vi "Init TS User Events.vi"(8 "error in (no error)":errorcluster, 11 "Generic Test Stand in":refnum<class "Generic Test Stand.lvclass">) -> (0 "error out":errorcluster, 3 "Generic Test Stand out":refnum<class "Generic Test Stand.lvclass">)   [LabVIEW 2019, in "Generic Test Stand.lvclass"]
uses:
  Generic Test Stand.lvclass
  Generic Test Stand.lvclass/Generic Test Stand.ctl
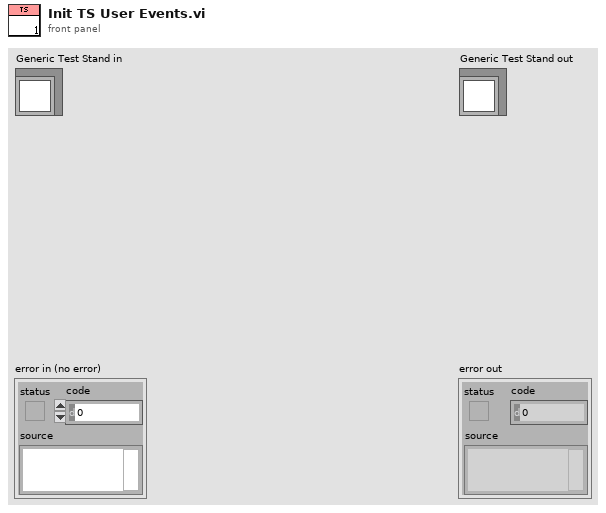
[diagram p1: front panel]
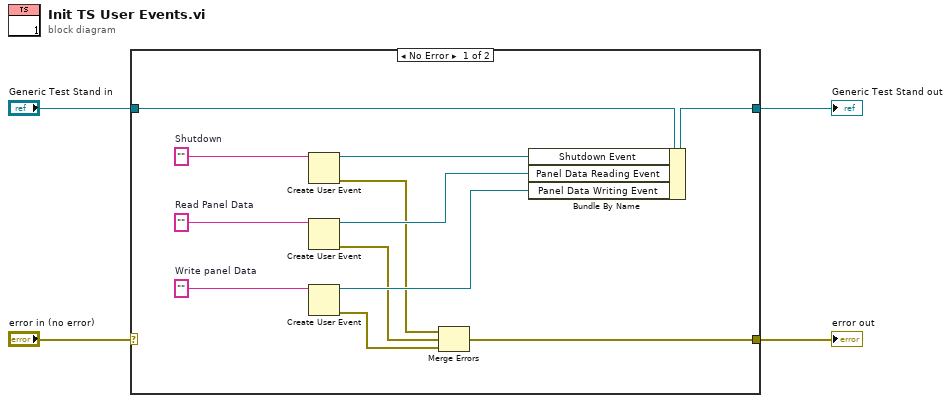
[diagram p0: block diagram]
diagram:
  n1 = case shown="No Error" "error in (no error)" {
    selector: "error in (no error)" -> [_ w18]
    tunnel: [w6 w18] -> w3
    tunnel: [w5 w17] -> w1
    tunnel: "Generic Test Stand in" -> [w13 w17]
    frame No Error {
      w14 = ""  # Write panel Data
      w15 = ""  # Read Panel Data
      w16 = ""  # Shutdown
      n2 = Create User Event(user event datatype=w16) -> (user event=w12:refnum<user-event>, error out=w9:errorcluster)  [unwired: 1 in]
      n3 = Create User Event(user event datatype=w15) -> (user event=w11:refnum<user-event>, error out=w8:errorcluster)  [unwired: 1 in]
      n4 = Create User Event(user event datatype=w14) -> (user event=w10:refnum<user-event>, error out=w7:errorcluster)  [unwired: 1 in]
      n5 = Merge Errors(w9, w8, w7) -> (w6:errorcluster)
      n6 = Bundle By Name(cluster=w13, "Shutdown Event"=w12, "Panel Data Reading Event"=w11, "Panel Data Writing Event"=w10) -> (w5:refnum<class "Generic Test Stand.lvclass">)
    }
    frame Error {
    }
  }
  "error out" <- w3
  "Generic Test Stand out" <- w1
